vi "Make_Triangles_from_Mapfile_PN.vi"(0 "XW_Calib_Map file path (dialog if empty)":path) -> (1 "XW_Calib_Map file path":path, 2 "Triangles":T1[](array[typedef]), 3 "Zero angle dataset from map (used for calib. correction)":dbl[][](array[numeric])=[[0.0, 0.0, 0.0, 0.0, 0.0], [0.0, 1.825705, 1.798205, 0.5414, 19.6], [0.0, 1.889865, 1.864295, 0.9965, 19.6], [0.0, 1.99866, 1.96829, 1.9949, 19.9], [0.0, 2.07712, 2.04351, 2.9915, 20.1], [0.0, 2.1396196, 2.104965, 4.0049, 20.1], [0.0, 2.191345, 2.155695, 5.0025, 20.1], [0.0, 2.275755, 2.2388, 6.9961, 20.1], [0.0, 2.34454, 2.306995, 9.0006, 20.1], [0.0, 2.40296, 2.365255, 11.0025, 20.1], [0.0, 2.45423, 2.4161, 12.9894, 20.3], [0.0, 2.50023, 2.462475, 15.0098, 20.3]] format="%0.3f")   [LabVIEW 2010]
uses:
  Triangle2D.ctl
  <vilib>/Utility/file.llb/Read From Spreadsheet File (string).vi
  <vilib>/Utility/file.llb/Read From Spreadsheet File (DBL).vi
panel:
  in  "Triangle2D":T1
  out "Quad centroids":T2(array[cluster])
  out "No. of quad. centroids":i32
  out "No. of triangles":i32
  out "Pts per set":i32
  out "Angle sets":i32
  out "Vertices (in AngleSets)":T3(array[cluster])
  in  "Vertex2D":cluster{"PosVector":dbl[], "ValueVector":dbl[]}
  out "all rows":string[][](array[string])
  # "Paul Nathan 12/12/09"
  # "17/02/10: Added calib. correction part.\n09/03/10: Changed angles to radians here to prevent calc. burden later"
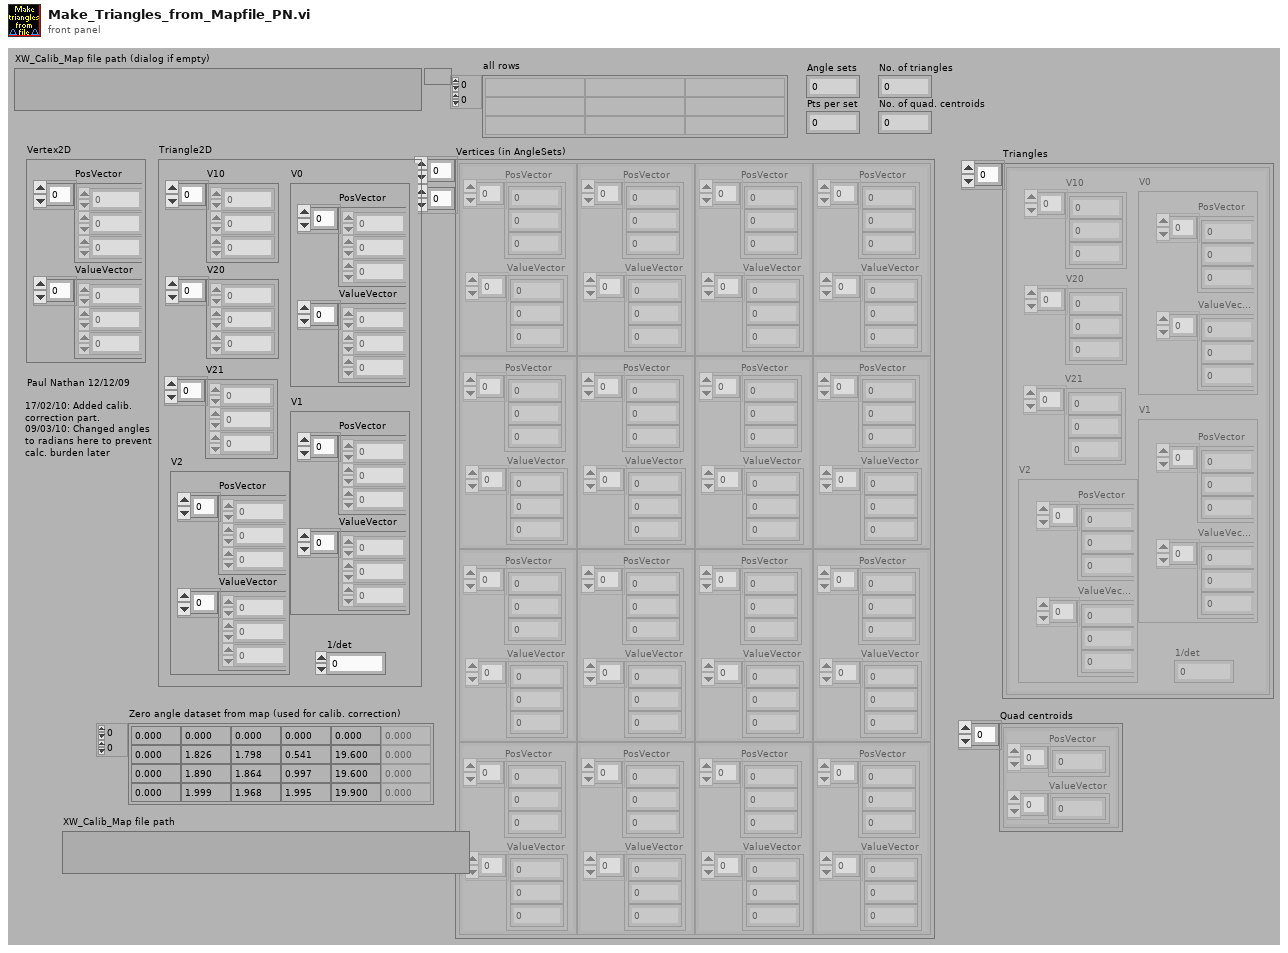
[diagram p1: front panel]
types:
  T1 = typedef "Triangle2D.ctl" = cluster{"V10":dbl[], "V20":dbl[], "1/det":dbl, "V0":cluster{"PosVector":dbl[], "ValueVector":dbl[]}, "V1":cluster{"PosVector":dbl[], "ValueVector":dbl[]}, "V2":cluster{"PosVector":dbl[], "ValueVector":dbl[]}, "V21":dbl[]}
  T2 = cluster{"PosVector":dbl[], "ValueVector":dbl[]}[]
  T3 = cluster{"PosVector":dbl[], "ValueVector":dbl[]}[][]
  T4 = cluster{"V10":dbl[], "V20":dbl[], "1/det":dbl, "V0":cluster{"PosVector":dbl[], "ValueVector":dbl[]}, "V1":cluster{"PosVector":dbl[], "ValueVector":dbl[]}, "V2":cluster{"PosVector":dbl[], "ValueVector":dbl[]}, "V21":dbl[]}
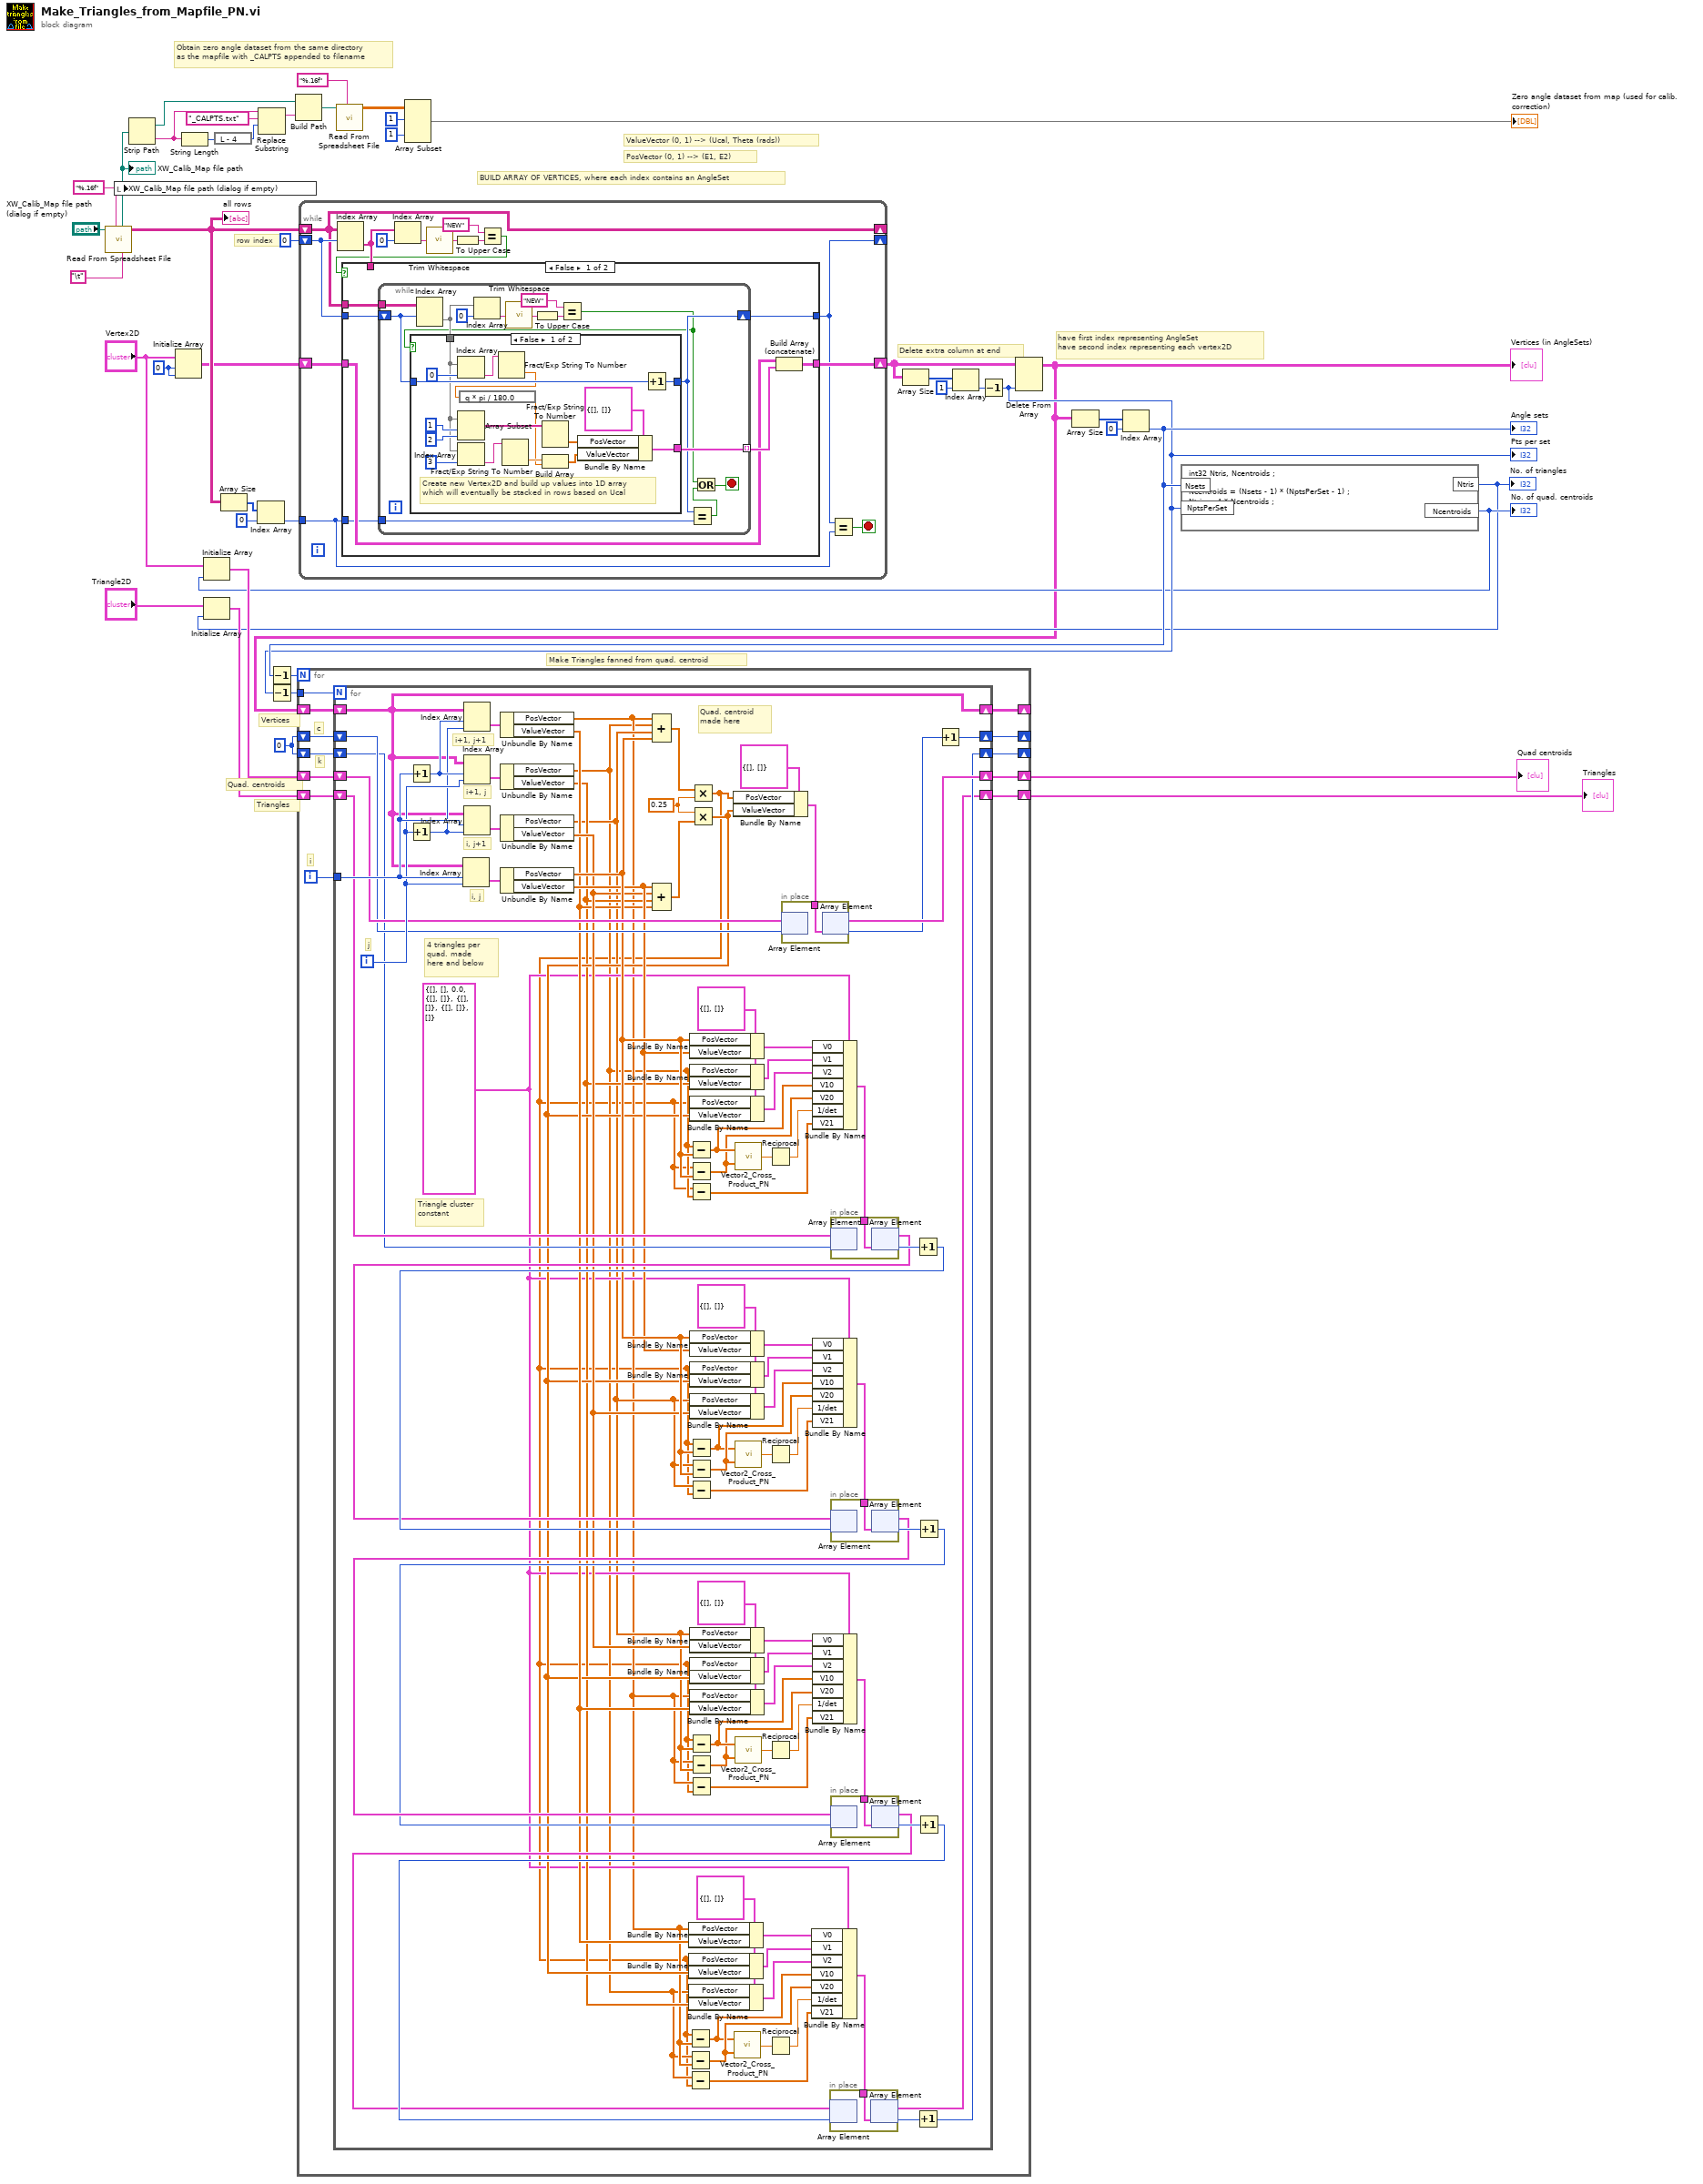
[diagram p0: block diagram]
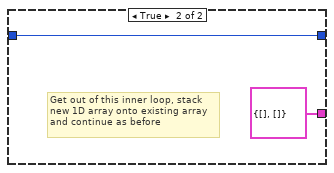
[diagram p2: hidden frame]
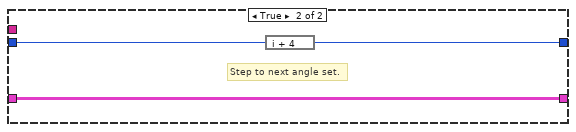
[diagram p3: hidden frame]
diagram:
  w31 = 0 ("index")
  w36 = 0 ("dimension size")
  # "Obtain zero angle dataset from the same directory as the mapfile with _CALPTS appended to filename"
  # "Make Triangles fanned from quad. centroid"
  # "Delete extra column at end"
  # "Triangles"
  # "Quad. centroids"
  # "Vertices"
  # "have first index representing AngleSet\nhave second index representing each vertex2D"
  # "BUILD ARRAY OF VERTICES, where each index contains an AngleSet"
  # "row index"
  # "PosVector (0, 1) --> (E1, E2)"
  # "ValueVector (0, 1) --> (Ucal, Theta (rads))"
  n1 = call-poly <vilib>:"Read From Spreadsheet File.vi"("delimiter (\\t)"="\t", "format (%s)"="%.16f" ("format (%.3f)"), "file path (dialog if empty)"="XW_Calib_Map file path (dialog if empty)") -> ("all rows"=w41:string[][], "new file path (Not A Path if cancelled)"=w4:path)  [unwired: 2 in, 5 out]
  "all rows" <- w41
  "XW_Calib_Map file path" <- w4
  n2 = local write "XW_Calib_Map file path (dialog if empty)"(w4) -> ()
  n3 = Strip Path(path=w4) -> (stripped path=w12:path, name=w16:string)
  n4 = Initialize Array("Vertex2D", w36, w36) -> (w35:T3)
  n5 = String Length(string=w16) -> (length=w15:i32)
  n6 = expression code="L - 4"(w15) -> (w14:i32)
  n7 = Array Size(array=w41) -> (size(s)=w38:i32[])
  n8 = Index Array(array=w38, index=0) -> (element=w37:i32)
  n9 = Replace Substring(3:w14, 4:"_CALPTS.txt" ("substring (\"\")"), 5:w16) -> (1:w11:string)  [unwired: 2 out]
  n10 = Build Path(base path=w12, name or relative path=w11) -> (appended path=w6:path)
  n11 = while {
    shift-right: [w49] -> w22
    shift-left: w35 -> [w50]
    shift-right: [w48] -> _
    shift-left: 0 ("index") -> [w53]
    tunnel: w37 -> [w47]
    shift-right: [w44] -> _
    shift-left: w41 -> [w44]
    stop <- w55 stop-if-true
    n12 = Index Array(array=w44, index (row)=w53) -> (element=w52:string[])  [unwired: 1 in]
    n13 = Index Array(array=w52, index=0) -> (element=w46:string)
    n14 = call <vilib>:"Trim Whitespace.vi"("string"=w46) -> ("trimmed string"=w45:string)  [unwired: 1 in]
    n15 = To Upper Case(1:w45) -> (0:w57:string)
    n16 = Equal?(x="NEW", y=w57) -> (x = y?=w51:bool)
    n17 = case shown="False" w51 {
      tunnel: w53 -> [w64 w100]
      tunnel: [w59 w98] -> w48
      tunnel: w52 -> [_ _]
      tunnel: w44 -> [w63 _]
      tunnel: w50 -> [w60 w99]
      tunnel: [w62 w99] -> w49
      tunnel: w47 -> [w58 _]
      frame False {
        n18 = while {
          tunnel: w63 -> [w74]
          shift-right: [w69] -> w59
          shift-left: w64 -> [w72]
          tunnel: [w73] -> w61 mode=indexing
          tunnel: w58 -> [w71]
          stop <- w68 stop-if-true
          n19 = Index Array(array=w74, index (row)=w72) -> (element=w75:string[])  [unwired: 1 in]
          n20 = Index Array(array=w75, index=0) -> (element=w66:string)
          n21 = call <vilib>:"Trim Whitespace.vi"("string"=w66) -> ("trimmed string"=w65:string)  [unwired: 1 in]
          n22 = To Upper Case(1:w65) -> (0:w78:string)
          n23 = Equal?(x="NEW", y=w78) -> (x = y?=w67:bool)
          n24 = case shown="False" w67 {
            tunnel: w75 -> [w84 _]
            tunnel: [w90 cluster{"PosVector":dbl[], "ValueVector":dbl[]} {"PosVector"=[], "ValueVector"=[]} ("Vertex2D")] -> w73
            tunnel: w72 -> [w89 w97]
            tunnel: [w88 w97] -> w69
            frame False {
              # "Create new Vertex2D and build up values into 1D array which will eventually be stacked in rows based on Ucal"
              n25 = Index Array(array=w84, index=0) -> (element=w93:string)
              n26 = Array Subset(array=w84, index=1, length=2) -> (w91:string[])
              n27 = Index Array(array=w84, index=3) -> (element=w82:string)
              n28 = Fract/Exp String To Number(string=w93) -> (number=w80:dbl)  [unwired: 1 in, 3 out]
              n29 = expression code="q * pi / 180.0"(w80) -> (w79:dbl)
              n30 = Fract/Exp String To Number(string=w82) -> (number=w83:dbl)  [unwired: 1 in, 3 out]
              n31 = Fract/Exp String To Number(string=w91) -> (number=w81:dbl[])  [unwired: 4 out]
              n32 = Build Array(w83, w79) -> (w95:dbl[])
              n33 = Bundle By Name(cluster=cluster{"PosVector":dbl[], "ValueVector":dbl[]} {"PosVector"=[], "ValueVector"=[]} ("Vertex2D"), "PosVector"=w81, "ValueVector"=w95) -> (w90:cluster{"PosVector":dbl[], "ValueVector":dbl[]})
              n34 = Increment(x=w89) -> (x+1=w88:i32)
            }
            frame True {
              # "Get out of this inner loop, stack new 1D array onto existing array and continue as before"
            }
          }
          n35 = Equal?(x=w69, y=w71) -> (x = y?=w70:bool)
          n36 = Or(x=w67, y=w70) -> (x .or. y?=w68:bool)
        }
        n37 = Build Array (concatenate)(w60, w61) -> (w62:T3)
      }
      frame True {
        # "Step to next angle set."
        n38 = expression code="i + 4"(w100) -> (w98:i32)
      }
    }
    n39 = Equal?(x=w48, y=w47) -> (x = y?=w55:bool)
  }
  n40 = call-poly <vilib>:"Read From Spreadsheet File.vi"("format (%.3f)"="%.16f", "file path (dialog if empty)"=w6) -> ("all rows"=w8:dbl[][])  [unwired: 2 in, 7 out]
  n41 = Array Subset(array=w8, index (row)=1 ("index"), index (col)=1 ("index")) -> (→"Zero angle dataset from map (used for calib. correction)":dbl[][])  [unwired: 2 in]
  n42 = Array Size(array=w22) -> (size(s)=w24:i32[])
  n43 = Index Array(array=w24, index=1) -> (element=w23:i32)
  n44 = Decrement(x=w23) -> (x-1=w20:i32)
  "Pts per set" <- w20
  n45 = Decrement(x=w20) -> (x-1=w29:i32)
  n46 = Delete From Array(array=w22, index (col)=w20) -> (array with subset deleted=w1:T3)  [unwired: 2 in, 1 out]
  "Vertices (in AngleSets)" <- w1
  n47 = Array Size(array=w1) -> (size(s)=w27:i32[])
  n48 = Index Array(array=w27, index=0) -> (element=w21:i32)
  "Angle sets" <- w21
  n49 = Decrement(x=w21) -> (x-1=w30:i32)
  n50 = formula code="int32 Ntris, Ncentroids ;\n\nNcentroids = (Nsets - 1) * (NptsPerSet - 1) ;\nNtris = 4 * Ncentroids ;"("Nsets"=w21, "NptsPerSet"=w20) -> ("Ntris"=w18:i32, "Ncentroids"=w19:i32)
  "No. of triangles" <- w18
  "No. of quad. centroids" <- w19
  n51 = Initialize Array("Vertex2D", w19) -> (w32:T2)
  n52 = Initialize Array("Triangle2D", w18) -> (w33:T1[])
  n53 = for {
    N: w30 -> [_]
    tunnel: w29 -> [w112]
    shift-right: [w106] -> _
    shift-left: w31 -> [w108]
    shift-right: [w105] -> _
    shift-left: w31 -> [w107]
    shift-right: [w103] -> w28
    shift-left: w32 -> [w109]
    shift-right: [w102] -> w2
    shift-left: w33 -> [w110]
    shift-right: [w101] -> _
    shift-left: w1 -> [w111]
    i -> [w104]
    # "i"
    # "k"
    # "c"
    n54 = for {
      N: w112 -> [_]
      shift-right: [w186] -> w106
      shift-left: w108 -> [w185]
      shift-right: [w136] -> w105
      shift-left: w107 -> [w180]
      tunnel: w104 -> [w196]
      shift-right: [w184] -> w103
      shift-left: w109 -> [w188]
      shift-right: [w135] -> w102
      shift-left: w110 -> [w181]
      shift-right: [w113] -> w101
      shift-left: w111 -> [w113]
      i -> [w195]
      w122 = T4 {"V10"=[], "V20"=[], "1/det"=0.0, "V0"={"PosVector"=[], "ValueVector"=[]}, "V1"={"PosVector"=[], "ValueVector"=[]}, "V2"={"PosVector"=[], "ValueVector"=[]}, "V21"=[]} ("Triangle2D")
      w141 = cluster{"PosVector":dbl[], "ValueVector":dbl[]} {"PosVector"=[], "ValueVector"=[]} ("Vertex2D")
      w155 = cluster{"PosVector":dbl[], "ValueVector":dbl[]} {"PosVector"=[], "ValueVector"=[]} ("Vertex2D")
      w164 = cluster{"PosVector":dbl[], "ValueVector":dbl[]} {"PosVector"=[], "ValueVector"=[]} ("Vertex2D")
      w175 = cluster{"PosVector":dbl[], "ValueVector":dbl[]} {"PosVector"=[], "ValueVector"=[]} ("Vertex2D")
      w189 = 0.25 ("x")
      # "4 triangles per quad. made here and below"
      # "Quad. centroid made here"
      # "Triangle cluster constant"
      # "i+1, j+1"
      # "i+1, j"
      # "i, j"
      # "i, j+1"
      # "j"
      n55 = Increment(x=w196) -> (x+1=w183:i32)
      n56 = Increment(x=w195) -> (x+1=w182:i32)
      n57 = Index Array(array=w113, index (row)=w196, index (col)=w195) -> (element=w194:cluster{"PosVector":dbl[], "ValueVector":dbl[]})
      n58 = Index Array(array=w113, index (row)=w183, index (col)=w182) -> (element=w191:cluster{"PosVector":dbl[], "ValueVector":dbl[]})
      n59 = Index Array(array=w113, index (row)=w183, index (col)=w195) -> (element=w192:cluster{"PosVector":dbl[], "ValueVector":dbl[]})
      n60 = Index Array(array=w113, index (row)=w196, index (col)=w182) -> (element=w193:cluster{"PosVector":dbl[], "ValueVector":dbl[]})
      n61 = Unbundle By Name(w191) -> ("PosVector"=w118:dbl[], "ValueVector"=w134:dbl[])
      n62 = Unbundle By Name(w192) -> ("PosVector"=w116:dbl[], "ValueVector"=w132:dbl[])
      n63 = Unbundle By Name(w193) -> ("PosVector"=w120:dbl[], "ValueVector"=w147:dbl[])
      n64 = Unbundle By Name(w194) -> ("PosVector"=w159:dbl[], "ValueVector"=w158:dbl[])
      n65 = Compound Arithmetic op=ADD(w118, w116, w120, w159) -> (w190:dbl[])
      n66 = Compound Arithmetic op=ADD(w158, w147, w132, w134) -> (w177:dbl[])
      n67 = Subtract(x=w116, y=w118) -> (x-y=w146:dbl[])
      n68 = Subtract(x=w116, y=w159) -> (x-y=w171:dbl[])
      n69 = Subtract(x=w120, y=w159) -> (x-y=w169:dbl[])
      n70 = Subtract(x=w118, y=w120) -> (x-y=w150:dbl[])
      n71 = Bundle By Name(cluster=w141, "PosVector"=w118, "ValueVector"=w134) -> (w142:cluster{"PosVector":dbl[], "ValueVector":dbl[]})
      n72 = Bundle By Name(cluster=w141, "PosVector"=w116, "ValueVector"=w132) -> (w144:cluster{"PosVector":dbl[], "ValueVector":dbl[]})
      n73 = Multiply(x=w190, y=w189) -> (x*y=w115:dbl[])
      n74 = Subtract(x=w115, y=w118) -> (x-y=w145:dbl[])
      n75 = Subtract(x=w116, y=w115) -> (x-y=w114:dbl[])
      n76 = Subtract(x=w115, y=w159) -> (x-y=w170:dbl[])
      n77 = Subtract(x=w115, y=w116) -> (x-y=w121:dbl[])
      n78 = Subtract(x=w115, y=w159) -> (x-y=w168:dbl[])
      n79 = Subtract(x=w120, y=w115) -> (x-y=w119:dbl[])
      n80 = Subtract(x=w115, y=w120) -> (x-y=w151:dbl[])
      n81 = Subtract(x=w118, y=w115) -> (x-y=w117:dbl[])
      n82 = Multiply(x=w189, y=w177) -> (x*y=w133:dbl[])
      n83 = Bundle By Name(cluster=w141, "PosVector"=w115, "ValueVector"=w133) -> (w143:cluster{"PosVector":dbl[], "ValueVector":dbl[]})
      n84 = Bundle By Name(cluster=w175, "PosVector"=w159, "ValueVector"=w158) -> (w174:cluster{"PosVector":dbl[], "ValueVector":dbl[]})
      n85 = Bundle By Name(cluster=w175, "PosVector"=w116, "ValueVector"=w132) -> (w173:cluster{"PosVector":dbl[], "ValueVector":dbl[]})
      n86 = Bundle By Name(cluster=w175, "PosVector"=w115, "ValueVector"=w133) -> (w172:cluster{"PosVector":dbl[], "ValueVector":dbl[]})
      n87 = Bundle By Name(cluster=w164, "PosVector"=w159, "ValueVector"=w158) -> (w165:cluster{"PosVector":dbl[], "ValueVector":dbl[]})
      n88 = Bundle By Name(cluster=w164, "PosVector"=w115, "ValueVector"=w133) -> (w166:cluster{"PosVector":dbl[], "ValueVector":dbl[]})
      n89 = Bundle By Name(cluster=w164, "PosVector"=w120, "ValueVector"=w147) -> (w167:cluster{"PosVector":dbl[], "ValueVector":dbl[]})
      n90 = Bundle By Name(cluster=w155, "PosVector"=w120, "ValueVector"=w147) -> (w154:cluster{"PosVector":dbl[], "ValueVector":dbl[]})
      n91 = Bundle By Name(cluster=w155, "PosVector"=w115, "ValueVector"=w133) -> (w153:cluster{"PosVector":dbl[], "ValueVector":dbl[]})
      n92 = Bundle By Name(cluster=w155, "PosVector"=w118, "ValueVector"=w134) -> (w152:cluster{"PosVector":dbl[], "ValueVector":dbl[]})
      n93 = Bundle By Name(cluster=cluster{"PosVector":dbl[], "ValueVector":dbl[]} {"PosVector"=[], "ValueVector"=[]} ("Vertex2D"), "PosVector"=w115, "ValueVector"=w133) -> (w187:cluster{"PosVector":dbl[], "ValueVector":dbl[]})
      n94 = call "Vector2_Cross_Product_PN.vi"("V (2D)"=w146, "U (2D)"=w145) -> ("U X V (2D)"=w124:dbl)
      n95 = call "Vector2_Cross_Product_PN.vi"("V (2D)"=w170, "U (2D)"=w171) -> ("U X V (2D)"=w130:dbl)
      n96 = call "Vector2_Cross_Product_PN.vi"("V (2D)"=w169, "U (2D)"=w168) -> ("U X V (2D)"=w128:dbl)
      n97 = call "Vector2_Cross_Product_PN.vi"("V (2D)"=w150, "U (2D)"=w151) -> ("U X V (2D)"=w126:dbl)
      n98 = Reciprocal(x=w130) -> (1/x=w129:dbl)
      n99 = Reciprocal(x=w128) -> (1/x=w127:dbl)
      n100 = Reciprocal(x=w126) -> (1/x=w125:dbl)
      n101 = Reciprocal(x=w124) -> (1/x=w123:dbl)
      n102 = in-place {
        in-place-border: w187 -> [w201]
        n103 = in-place-array #1(w188, w185) -> ()  [unwired: 1 out]
        n104 = in-place-array #1(w201) -> (w184:T2, w131:i32)
      }
      n105 = Bundle By Name(cluster=w122, "V0"=w142, "V1"=w143, "V2"=w144, "V10"=w145, "V20"=w146, "1/det"=w123, "V21"=w114) -> (w139:T4)
      n106 = Bundle By Name(cluster=w122, "V0"=w174, "V1"=w173, "V2"=w172, "V10"=w171, "V20"=w170, "1/det"=w129, "V21"=w121) -> (w179:T4)
      n107 = Bundle By Name(cluster=w122, "V0"=w165, "V1"=w166, "V2"=w167, "V10"=w168, "V20"=w169, "1/det"=w127, "V21"=w119) -> (w162:T4)
      n108 = Bundle By Name(cluster=w122, "V0"=w154, "V1"=w153, "V2"=w152, "V10"=w151, "V20"=w150, "1/det"=w125, "V21"=w117) -> (w157:T4)
      n109 = in-place {
        in-place-border: w179 -> [w200]
        n110 = in-place-array #2(w181, w180) -> ()  [unwired: 1 out]
        n111 = in-place-array #2(w200) -> (w160:T1[], w178:i32)
      }
      n112 = Increment(x=w178) -> (x+1=w161:i32)
      n113 = in-place {
        in-place-border: w162 -> [w199]
        n114 = in-place-array #3(w160, w161) -> ()  [unwired: 1 out]
        n115 = in-place-array #3(w199) -> (w149:T1[], w163:i32)
      }
      n116 = Increment(x=w163) -> (x+1=w148:i32)
      n117 = in-place {
        in-place-border: w157 -> [w198]
        n118 = in-place-array #4(w149, w148) -> ()  [unwired: 1 out]
        n119 = in-place-array #4(w198) -> (w137:T1[], w156:i32)
      }
      n120 = Increment(x=w156) -> (x+1=w138:i32)
      n121 = in-place {
        in-place-border: w139 -> [w197]
        n122 = in-place-array #5(w137, w138) -> ()  [unwired: 1 out]
        n123 = in-place-array #5(w197) -> (w135:T1[], w140:i32)
      }
      n124 = Increment(x=w140) -> (x+1=w136:i32)
      n125 = Increment(x=w131) -> (x+1=w186:i32)
    }
  }
  "Quad centroids" <- w28
  "Triangles" <- w2
